vi "Get Legend Display.vi"(6 "Control Ref Queue":T1, 8 "error in (no error)":errorcluster, 9 "Active Plot":i32, 10 "Plot Name":string[](array[string]), 11 "Color Pair Array":cluster{"Color":u32, "String":string}[](array[cluster])) -> (0 "error out":errorcluster, 1 "Ignore the size change?":bool)   [LabVIEW 2017, in "3D Plot.lvclass"]
uses:
  <vilib>/Math Plots/3D Math Plots/3D Plot/3D Plot/3D Plot.lvclass
  <vilib>/Math Plots/3D Math Plots/3D Plot/Action String/3DMathPlot Ctrl Act Queue.ctl
  <vilib>/Math Plots/3D Math Plots/3D Plot/Action String/3DMathPlot Ctrl Act Cluster.ctl
  <vilib>/Math Plots/3D Math Plots/3D Plot/Action String/3DMathPlot State Class.ctl
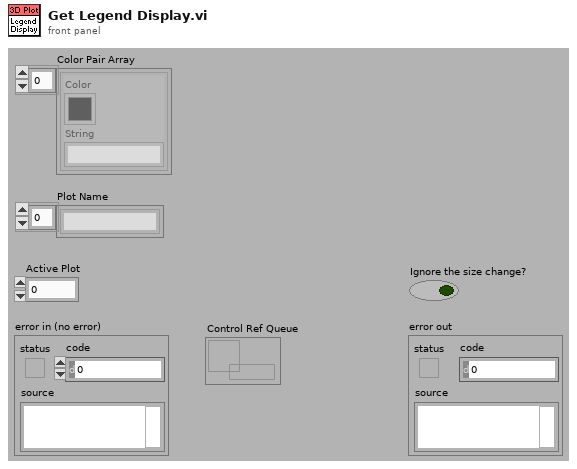
[diagram p1: front panel]
types:
  T1 = typedef "3DMathPlot Ctrl Act Queue.ctl" = refnum<queue>
  T2 = enum16{"User-specified Font", "Application Font", "System Font", "Dialog Font"}
  T3 = typedef "3DMathPlot Ctrl Act Cluster.ctl" = cluster{"3D Picture Control":refnum<vi>, "Render Window Refnum":refnum<vi>, "XY Graph":refnum<vi>, "Intensity Graph":refnum<vi>, "Color Legend Palette":refnum<vi>, "Projection Palette":refnum<vi>, "XControl  Ref":refnum<vi>, "Facade Ref":refnum<vi>, "Export Image Ref":refnum<vi>, "Clear Data Flag":bool, "Display State Change Class":T4}
  T4 = typedef "3DMathPlot State Class.ctl" = enum16{"Update All Objects (Undo)", "Update Light Object Only", "Update Axis Object Only", "Update Plot Object Only", "Update Cursor Object Only", "Update Axis Plot Cursor Objects", "No Update"}
  T5 = cluster{"left":i16, "top":i16, "right":i16, "bottom":i16}
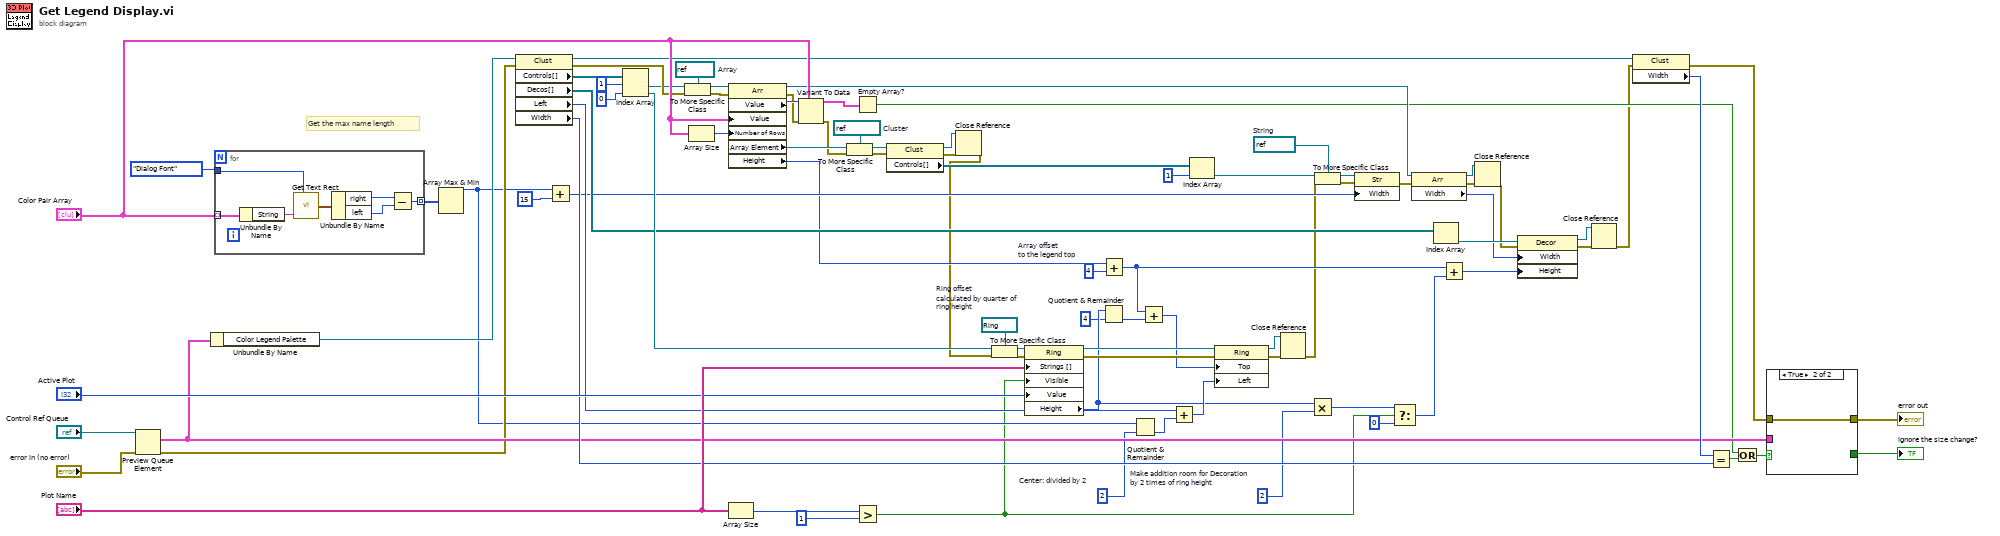
[diagram p0: block diagram]
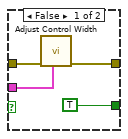
[diagram p2: hidden frame]
diagram:
  w23 = u32 4  # Ring offset calculated by quarter of ring height
  w24 = u32 4  # Array offset to the legend top
  w30 = u32 2  # Make addition room for Decoration by 2 times of ring height
  w37 = i16 2  # Center: divided by 2
  w64 = refnum<vi> refnum  # String
  w59 = refnum<vi> refnum  # Cluster
  w54 = refnum<vi> refnum  # Array
  # "Get the max name length"
  n1 = Preview Queue Element(queue="Control Ref Queue", error in (no error)="error in (no error)") -> (element=w41:T3, error out=w39:errorcluster)  [unwired: 3 out]
  n2 = Unbundle By Name(w41) -> ("Color Legend Palette"=w80:refnum<vi>)
  n3 = for {
    tunnel: "Color Pair Array" -> [w94] mode=indexing
    tunnel: [w89] -> w57 mode=indexing
    tunnel: T2."Dialog Font" ("desired font(Application)") -> [w88]
    n4 = Unbundle By Name(w94) -> ("String"=w90:string)
    n5 = call <vilib>:"Get Text Rect.vi"("desired font(Application)"=w88, "text"=w90) -> ("rect"=w93:T5)  [unwired: 4 in, 3 out]
    n6 = Unbundle By Name(w93) -> ("right"=w92:i16, "left"=w91:i16)
    n7 = Subtract(x=w92, y=w91) -> (x-y=w89:i16)
  }
  n8 = Array Max & Min(array=w57) -> (max value=w35:i16)  [unwired: 3 out]
  n9 = property class="Clust"(reference=w80, error in=w39) -> (reference out=w45:refnum<vi>, error out=w74:errorcluster, "Controls[]"=w51:refnum<vi>[], "Decos[]"=w50:refnum<vi>[], "Left"=w40:i32, "Width"=w43:u32)
  n10 = Add(x=w35, y=u32 15) -> (x+y=w36:u32)
  n11 = Index Array(array=w51, index #1=1 ("index"), index #2=0 ("index")) -> (element #1=w53:refnum<vi>, element #2=w77:refnum<vi>)
  n12 = To More Specific Class(target class=w54, reference=w53, error in=w74) -> (specific class reference=w56:refnum<vi>, error out=w55:errorcluster)
  n13 = Array Size(array="Color Pair Array") -> (size(s)=w68:i32)
  n14 = property class="Arr"(reference=w56, error in=w55, "Value"="Color Pair Array", "Number of Rows"=w68) -> (reference out=w28:refnum<vi>, error out=w13:errorcluster, "Value"=w19:variant, "Array Element"=w58:refnum<vi>, "Height"=w32:u32)
  n15 = Array Size(array="Plot Name") -> (size(s)=w22:i32)
  n16 = Variant To Data(error in=w13, type="Color Pair Array", Variant=w19) -> (data=w18:cluster{"Color":u32, "String":string}[], error out=w14:errorcluster)
  n17 = To More Specific Class(target class=w59, reference=w58, error in=w14) -> (specific class reference=w60:refnum<vi>, error out=w75:errorcluster)
  n18 = Empty Array?(array=w18) -> (empty?=w17:bool)
  n19 = Greater?(x=w22, y=1) -> (0:w20:bool)
  n20 = property class="Clust"(reference=w60, error in=w75) -> (reference out=w6:refnum<vi>, error out=w5:errorcluster, "Controls[]"=w62:refnum<vi>[])
  n21 = Close Reference(reference=w6, error in (no error)=w5) -> (error out=w4:errorcluster)
  n22 = To More Specific Class(target class=refnum<vi> refnum ("specific class reference"), reference=w77, error in=w4) -> (specific class reference=w70:refnum<vi>, error out=w69:errorcluster)
  n23 = property class="Ring"(reference=w70, error in=w69, "Strings []"="Plot Name", "Visible"=w20, "Value"="Active Plot") -> (reference out=w47:refnum<vi>, error out=w46:errorcluster, "Height"=w31:u32)
  n24 = Add(x=w32, y=w24) -> (x+y=w25:u32)
  n25 = Quotient & Remainder(x=w31, y=w23) -> (floor(x/y)=w34:u32)  [unwired: 1 out]
  n26 = Quotient & Remainder(x=w35, y=w37) -> (floor(x/y)=w49:i16)  [unwired: 1 out]
  n27 = Add(x=w25, y=w34) -> (x+y=w33:u32)
  n28 = Add(x=w40, y=w49) -> (x+y=w48:i32)
  n29 = Index Array(array=w62, index=1) -> (element=w65:refnum<vi>)
  n30 = property class="Ring"(reference=w47, error in=w46, "Top"=w33, "Left"=w48) -> (reference out=w3:refnum<vi>, error out=w2:errorcluster)
  n31 = Close Reference(reference=w3, error in (no error)=w2) -> (error out=w1:errorcluster)
  n32 = Multiply(x=w31, y=w30) -> (x*y=w29:u32)
  n33 = To More Specific Class(target class=w64, reference=w65, error in=w1) -> (specific class reference=w63:refnum<vi>, error out=w78:errorcluster)
  n34 = property class="Str"(reference=w63, error in=w78, "Width"=w36) -> (error out=w27:errorcluster)  [unwired: 1 out]
  n35 = Select(t=w29, s=w20, f=u32 0 ("x")) -> (s? t:f=w73:u32)
  n36 = property class="Arr"(reference=w28, error in=w27) -> (reference out=w12:refnum<vi>, error out=w11:errorcluster, "Width"=w26:u32)
  n37 = Index Array(array=w50) -> (element=w67:refnum<vi>)  [unwired: 1 in]
  n38 = Add(x=w25, y=w73) -> (x+y=w79:u32)
  n39 = Close Reference(reference=w12, error in (no error)=w11) -> (error out=w10:errorcluster)
  n40 = property class="Decor"(reference=w67, error in=w10, "Width"=w26, "Height"=w79) -> (reference out=w9:refnum<vi>, error out=w8:errorcluster)
  n41 = Close Reference(reference=w9, error in (no error)=w8) -> (error out=w7:errorcluster)
  n42 = property class="Clust"(reference=w45, error in=w7) -> (error out=w42:errorcluster, "Width"=w44:u32)  [unwired: 1 out]
  n43 = Equal?(x=w44, y=w43) -> (x = y?=w16:bool)
  n44 = Or(x=w17, y=w16) -> (x .or. y?=w15:bool)
  n45 = case shown="True" w15 {
    tunnel: [w98 w99] -> w85
    tunnel: w41 -> [w97 _]
    tunnel: [TRUE _] -> w87
    tunnel: w42 -> [w95 w99]
    frame False {
      n46 = call <vilib>:"Adjust Control Width.vi"("Control Ref Cluster"=w97, "error in (no error)"=w95) -> ("error out"=w98:errorcluster)  [unwired: 6 in, 3 out]
    }
    frame True {
    }
  }
  "Ignore the size change?" <- w87
  "error out" <- w85
